vi "DeMod6.vi"(9 "State":dbl, 11 "Steps":i32) -> (3 "Numeric out":i32)   [LabVIEW 2020]
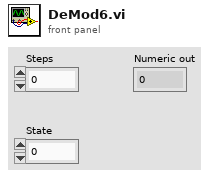
[diagram p1: front panel]
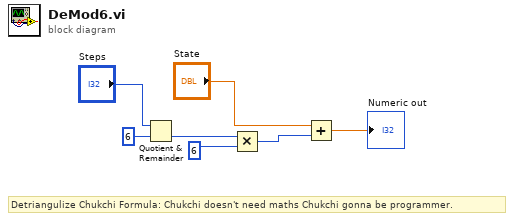
[diagram p0: block diagram]
diagram:
  # "Detriangulize Chukchi Formula: Chukchi doesn't need maths Chukchi gonna be programmer."
  n1 = Quotient & Remainder(x="Steps", y=6) -> (floor(x/y)=w4:i32)  [unwired: 1 out]
  n2 = Multiply(x=w4, y=6) -> (x*y=w6:i32)
  n3 = Add(x="State", y=w6) -> (x+y=→"Numeric out":dbl)
